vi "digital_line_cycler.vi"() -> ()   [LabVIEW 2012]
uses:
  <vilib>/DAQmx/write.llb/DAQmx Write (Digital Wfm 1Chan NSamp).vi
  <vilib>/Waveform/DWDTOps.llb/Digital Pattern Generator (Single Value).vi
  <vilib>/DAQmx/create/channels.llb/DAQmx Create Channel (DO-Digital Output).vi
  <vilib>/Waveform/DWDTOps.llb/DWDT Append Digital Samples.vi
  <vilib>/Waveform/DWDTOps.llb/DWDT Digital Size.vi
  <vilib>/DAQmx/configure/timing.llb/DAQmx Timing (Sample Clock).vi
  <vilib>/Waveform/DWDTOps.llb/DWDT Uncompress Digital.vi
  <vilib>/DAQmx/miscellaneous.llb/DAQmx Fill In Error Info.vi
  <resource>/objmgr/daqmx.rc
panel:
  in  "error in":errorcluster
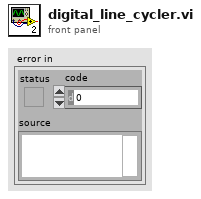
[diagram p1: front panel]
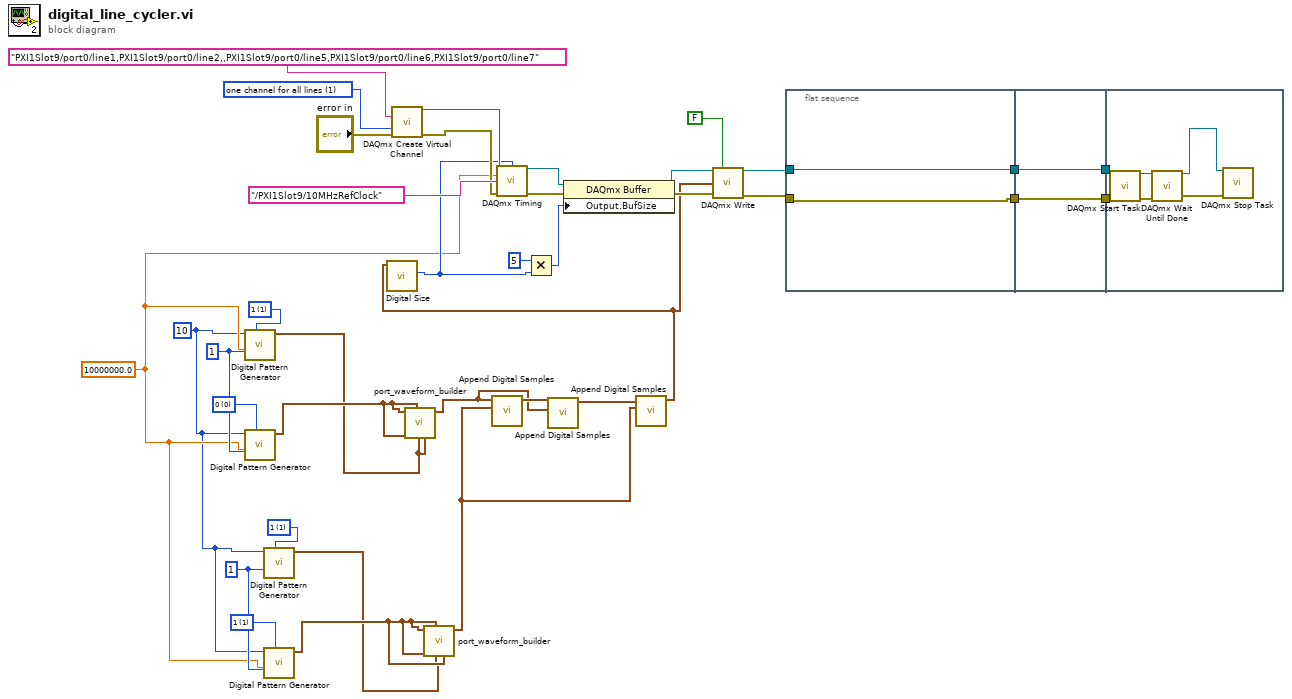
[diagram p0: block diagram]
diagram:
  w13 = u8 1 items=["0", "1", "Z", "L", "H", "X", "T", "V"] ("value")
  w14 = u32 1 ("number of signals")
  w10 = u8 1 items=["0", "1", "Z", "L", "H", "X", "T", "V"] ("value")
  w17 = u8 0 items=["0", "1", "Z", "L", "H", "X", "T", "V"] ("value")
  w22 = u32 1 ("number of signals")
  w3 = u32 10 ("number of samples")
  w23 = u8 1 items=["0", "1", "Z", "L", "H", "X", "T", "V"] ("value")
  w27 = 1 items=["one channel for each line", "one channel for all lines"] ("line grouping")
  w9 = 10000000.0 ("rate")
  n1 = call-poly <vilib>:"Digital Pattern Generator.vi"("value"=w23, "sample rate"=w9, "number of signals"=w22, "number of samples"=w3) -> ("digital waveform"=w1:digitalwaveform)  [unwired: 6 in, 1 out]
  n2 = call-poly <vilib>:"Digital Pattern Generator.vi"("value"=w17, "sample rate"=w9, "number of signals"=w22, "number of samples"=w3) -> ("digital waveform"=w2:digitalwaveform)  [unwired: 6 in, 1 out]
  n3 = call-poly <vilib>:"Digital Pattern Generator.vi"("value"=w10, "number of signals"=w14, "number of samples"=w3) -> ("digital waveform"=w11:digitalwaveform)  [unwired: 7 in, 1 out]
  n4 = call-poly <vilib>:"Digital Pattern Generator.vi"("value"=w13, "sample rate"=w9, "number of signals"=w14, "number of samples"=w3) -> ("digital waveform"=w12:digitalwaveform)  [unwired: 6 in, 1 out]
  n5 = call-poly <vilib>:"DAQmx Create Virtual Channel.vi"("lines"=tag "PXI1Slot9/port0/line1,PXI1Slot9/port0/line2,,PXI1Slot9/port0/line5,PXI1Slot9/port0/line6,PXI1Slot9/port0/line7", "line grouping"=w27, "error in"="error in") -> ("task out"=w28:refnum<k21>, "error out"=w25:errorcluster)  [unwired: 11 in]
  n6 = call "port_waveform_builder.vi"("Line 7"=w1, "Line 6"=w1, "Line 1"=w2, "Line 5"=w2, "Line 2"=w2) -> ("digital waveform out"=w7:digitalwaveform)  [unwired: 6 in]
  n7 = call "port_waveform_builder.vi"("Line 7"=w12, "Line 6"=w11, "Line 1"=w12, "Line 5"=w12, "Line 2"=w12) -> ("digital waveform out"=w5:digitalwaveform)  [unwired: 6 in]
  n8 = call-poly <vilib>:"Append Digital Samples.vi"("digital waveform B"=w5, "digital waveform A"=w7) -> ("digital waveform out"=w8:digitalwaveform)  [unwired: 8 in, 1 out]
  n9 = call-poly <vilib>:"Append Digital Samples.vi"("digital waveform B"=w7, "digital waveform A"=w8) -> ("digital waveform out"=w6:digitalwaveform)  [unwired: 8 in, 1 out]
  n10 = call-poly <vilib>:"Append Digital Samples.vi"("digital waveform B"=w5, "digital waveform A"=w6) -> ("digital waveform out"=w4:digitalwaveform)  [unwired: 8 in, 1 out]
  n11 = call-poly <vilib>:"Digital Size.vi"("digital waveform in"=w4) -> ("number of samples"=w18:i32)  [unwired: 7 in, 3 out]
  n12 = call-poly <vilib>:"DAQmx Timing.vi"("task/channels in"=w28, "samples per channel"=w18, "rate"=w9, "source"=tag "/PXI1Slot9/10MHzRefClock", "error in"=w25) -> ("task out"=w32:refnum<k21>, "error out"=w31:errorcluster)  [unwired: 9 in]
  n13 = Multiply(x=5, y=w18) -> (x*y=w19:i32)
  n14 = property class="DAQmx Buffer"(reference=w32, error in=w31, "Output.BufSize"=w19) -> (reference out=w29:refnum<k21>, error out=w24:errorcluster)
  n15 = call-poly <vilib>:"DAQmx Write.vi"("task/channels in"=w29, "auto start"=FALSE, "data"=w4, "error in"=w24) -> ("task out"=w15:refnum<k21>, "error out"=w16:errorcluster)  [unwired: 9 in, 1 out]
  n16 = flat-sequence {
    tunnel: w16 -> [w38]
    tunnel: w15 -> [w39]
    tunnel: [w39] -> w37
    tunnel: [w38] -> w36
    tunnel: w37 -> [w41]
    tunnel: [w41] -> w35
    tunnel: [w40] -> w34
    tunnel: w36 -> [w40]
    tunnel: w35 -> [w47]
    tunnel: w34 -> [w46]
    frame #0 {
    }
    frame #1 {
    }
    frame #2 {
      n17 = call <vilib>:"DAQmx Start Task.vi"("task/channels in"=w47, "error in"=w46) -> ("task out"=w44:refnum<k21>, "error out"=w45:errorcluster)  [unwired: 12 in]
      n18 = call <vilib>:"DAQmx Wait Until Done.vi"("task/channels in"=w44, "error in"=w45) -> ("task out"=w42:refnum<k21>, "error out"=w43:errorcluster)  [unwired: 12 in]
      n19 = call <vilib>:"DAQmx Stop Task.vi"("task/channels in"=w42, "error in"=w43) -> ()  [unwired: 12 in, 2 out]
    }
  }
